vi "LSMcontroller_v62_updatedpointscan.vi"() -> ()   [LabVIEW 2015] (continued)
                                tunnel: [w2766 w2779] -> w2756
                                tunnel: w2760 -> [w2775 w2794]
                                tunnel: w2761 -> [w2765 w2785]
                                tunnel: w2762 -> [_ w2791]
                                frame False {
                                w2769 = u16 0 items=["unsigned binary", "offset binary", "2's complement"] ("data format (offset binary)")
                                n482 = Initialize Array(sgl 0.0, w2765) -> (w2772:sgl[])
                                n483 = Replace Array Subset(array=w2772, new element=sgl 1.0, index=0) -> (w2770:sgl[])
                                n484 = Reciprocal(x=w2775) -> (1/x=w2776:sgl)
                                n485 = Bundle By Name("Y"=w2770, "dt"=w2776) -> (w2767:waveform(sgl))  [unwired: 1 in]
                                n486 = call-poly <vilib>:"Analog to Digital.vi"("data format (offset binary)"=w2769, "compress digital (T)"=TRUE, "full-scale range (pk-pk)"=1.0, "resolution (16 bit)"=1, "analog waveform"=w2767) -> ("digital waveform"=w2766:digitalwaveform)  [unwired: 3 in, 3 out]
                                }
                                frame True {
                                w2782 = u16 0 items=["unsigned binary", "offset binary", "2's complement"] ("data format (offset binary)")
                                n487 = To Double Precision Float(number=w2785) -> (double precision float=w2792:dbl)
                                n488 = Initialize Array(sgl 0.0, w2785) -> (w2787:sgl[])
                                n489 = Divide(x=w2791, y=w2792) -> (x/y=w2789:dbl)
                                n490 = Round Toward +Infinity(x=w2789) -> (ceil(x): smallest int >= x=w2790:dbl)
                                n491 = Replace Array Subset(array=w2787, new element=sgl 1.0, index=0) -> (w2784:sgl[])
                                n492 = for {
                                N: w2790 -> [_]
                                tunnel: w2784 -> [w2796]
                                tunnel: [w2796] -> w2793 mode=concatenating
                                }
                                n493 = Reciprocal(x=w2794) -> (1/x=w2795:sgl)
                                n494 = Bundle By Name("Y"=w2793, "dt"=w2795) -> (w2780:waveform(sgl))  [unwired: 1 in]
                                n495 = call-poly <vilib>:"Analog to Digital.vi"("data format (offset binary)"=w2782, "compress digital (T)"=TRUE, "full-scale range (pk-pk)"=1.0, "resolution (16 bit)"=1, "analog waveform"=w2780) -> ("digital waveform"=w2779:digitalwaveform)  [unwired: 3 in, 3 out]
                                }
                                }
                                n496 = Build Array (concatenate)(w2754, w2756) -> (w2752:digitalwaveform[])
                                n497 = call "waveformsDObuffer.vi"("DO wf in"=w2752, "command"="set") -> ()  [unwired: 1 out]
                                }
                                frame 2 {
                                n498 = call "waveformsDObuffer.vi"("command"="get") -> ("DO wf out"=w2800:digitalwaveform[])  [unwired: 1 in]
                                n499 = Delete From Array(array=w2800, length=1, index=w2803) -> (deleted portion=w2798:digitalwaveform[], array with subset deleted=w2797:digitalwaveform[])
                                n500 = call "waveformsDObuffer.vi"("DO wf in"=w2797, "command"="set") -> ()  [unwired: 1 out]
                                }
                                frame 3, Default {
                                }
                                frame 0 {
                                n501 = local read "Measurement"() -> (w2806:T4)
                                n502 = To Unsigned Long Integer(number=w2806) -> (unsigned 32bit integer=w2805:u32)
                                n503 = case shown="5..7" w2805 {
                                tunnel: w2807 -> [_ w2810]
                                tunnel: [_ w2809] -> w2804
                                frame 0..4, Default {
                                }
                                frame 5..7 {
                                n504 = call "2pparameters.vi"("command"="get") -> ("params out"=w2817:T10)  [unwired: 1 in]
                                n505 = Unbundle By Name(w2817) -> ("wavdet"=w2818:bool, "sAOxy"=w2820:i32, "refwfsize"=w2821:dbl, "srate Img"=w2819:sgl)
                                n506 = call "waveformsDObuffer.vi"("command"="get") -> ("DO wf out"=w2811:digitalwaveform[])  [unwired: 1 in]
                                n507 = Index Array(array=w2811, index=w2810) -> (element=w2812:digitalwaveform)
                                n508 = case shown="True" w2818 {
                                tunnel: [w2825 w2838] -> w2815
                                tunnel: w2819 -> [w2834 w2853]
                                tunnel: w2820 -> [w2824 w2844]
                                tunnel: w2821 -> [_ w2850]
                                frame False {
                                w2828 = u16 0 items=["unsigned binary", "offset binary", "2's complement"] ("data format (offset binary)")
                                n509 = Initialize Array(sgl 0.0, w2824) -> (w2831:sgl[])
                                n510 = Replace Array Subset(array=w2831, new element=sgl 1.0, index=0) -> (w2829:sgl[])
                                n511 = Reciprocal(x=w2834) -> (1/x=w2835:sgl)
                                n512 = Bundle By Name("Y"=w2829, "dt"=w2835) -> (w2826:waveform(sgl))  [unwired: 1 in]
                                n513 = call-poly <vilib>:"Analog to Digital.vi"("data format (offset binary)"=w2828, "compress digital (T)"=TRUE, "full-scale range (pk-pk)"=1.0, "resolution (16 bit)"=1, "analog waveform"=w2826) -> ("digital waveform"=w2825:digitalwaveform)  [unwired: 3 in, 3 out]
                                }
                                frame True {
                                w2841 = u16 0 items=["unsigned binary", "offset binary", "2's complement"] ("data format (offset binary)")
                                n514 = To Double Precision Float(number=w2844) -> (double precision float=w2851:dbl)
                                n515 = Initialize Array(sgl 0.0, w2844) -> (w2846:sgl[])
                                n516 = Divide(x=w2850, y=w2851) -> (x/y=w2848:dbl)
                                n517 = Round Toward +Infinity(x=w2848) -> (ceil(x): smallest int >= x=w2849:dbl)
                                n518 = Replace Array Subset(array=w2846, new element=sgl 1.0, index=0) -> (w2843:sgl[])
                                n519 = for {
                                N: w2849 -> [_]
                                tunnel: w2843 -> [w2855]
                                tunnel: [w2855] -> w2852 mode=concatenating
                                }
                                n520 = Reciprocal(x=w2853) -> (1/x=w2854:sgl)
                                n521 = Bundle By Name("Y"=w2852, "dt"=w2854) -> (w2839:waveform(sgl))  [unwired: 1 in]
                                n522 = call-poly <vilib>:"Analog to Digital.vi"("data format (offset binary)"=w2841, "compress digital (T)"=TRUE, "full-scale range (pk-pk)"=1.0, "resolution (16 bit)"=1, "analog waveform"=w2839) -> ("digital waveform"=w2838:digitalwaveform)  [unwired: 3 in, 3 out]
                                }
                                }
                                n523 = Build Array(w2812) -> (w2809:digitalwaveform[])
                                n524 = Replace Array Subset(array=w2811, new element=w2815, index=w2810) -> (w2808:digitalwaveform[])
                                n525 = call "waveformsDObuffer.vi"("DO wf in"=w2808, "command"="set") -> ()  [unwired: 1 out]
                                }
                                }
                                }
                                }
                              }
                              frame #10 {
                                n526 = local read "Meastab"() -> (w2870:enum32{"X-Y Image", "Linescan", "Timetrace"})
                                n527 = property on="refwf" class="Ring (strict)"() -> ("RingText.Text"=w2867:string)  [unwired: 2 in, 2 out]
                                n528 = case shown="\"Timetrace\"" w2870 {
                                tunnel: [w2872 w2873] -> w2871
                                frame "X-Y Image", Default {
                                n529 = local read "Sampling rate"() -> (w2872:dbl)
                                }
                                frame "Timetrace" {
                                n530 = local read "srateAODOtt"() -> (w2873:dbl)
                                }
                                }
                                n531 = call "waveformsAObuffer.vi"("command"="get") -> ("AO wf out"=w2858:waveform(dbl)[])  [unwired: 1 in]
                                n532 = local read "wavdet"() -> (w2868:bool)
                                n533 = call "waveformsDObuffer.vi"("command"="get") -> ("DO wf out"=w2862:digitalwaveform[])  [unwired: 1 in]
                                n534 = call "correctwaveformsizetemp.vi"("new sampling frequency (Hz)"=w2871, "start"=TRUE, "reference waveforms to"=w2867, "Analog waveforms in"=w2858, "stop"=FALSE, "Digital waveforms in"=w2862) -> ("analog wf out"=w2864:waveform(dbl)[], "Digital wf out"=w2866:digitalwaveform[], "measpoints"=w2869:i32)
                                n535 = call "GetNumCamFramesv2.vi"("Digital Waveform Graph"=w2866) -> ("Numeric"=w2865:i32)  [unwired: 10 in]
                                n536 = call "waveformsDObuffer.vi"("DO wf in"=w2866, "command"="set") -> ()  [unwired: 1 out]
                                n537 = call "waveformsAObuffer.vi"("AO wf in"=w2864, "command"="set") -> ()  [unwired: 1 out]
                                n538 = local write "Total Camera Frames"(w2865) -> ()
                                n539 = case shown="True" w2868 {
                                tunnel: w2869 -> [_ w2874]
                                frame False {
                                }
                                frame True {
                                n540 = local write "# of frames"(w2874) -> ()
                                }
                                }
                              }
                            }
                          }
                          frame #6 {
                            # "Disabled for conversion to 64 bit"
                            n541 = disable-structure shown="Disabled" {
                              frame Disabled {
                                n542 = local read "Measurement"() -> (w2879:T4)
                                n543 = case shown="\"Lifetime (scan)\"" w2879 {
                                frame "X-Y-t movie", Default {
                                }
                                frame "Lifetime (scan)" {
                                # "total acquisition time"
                                n544 = call "2pparameters.vi"("command"="get") -> ("params out"=w2885:T10)  [unwired: 1 in]
                                n545 = Unbundle By Name(w2885) -> ("measpoints"=w2906:i32, "avpp"=w2907:i32, "sAOxy"=w2886:i32, "srate Img"=w2908:sgl)
                                n546 = Multiply(x=w2906, y=w2907) -> (x*y=w2904:i32)
                                n547 = To Double Precision Float(number=w2886) -> (double precision float=w2891:dbl)
                                n548 = Divide(x=w2891, y=w2908) -> (x/y=w2893:dbl)
                                n549 = To Double Precision Float(number=w2904) -> (double precision float=w2889:dbl)
                                n550 = local read "min phot"() -> (w2900:u32)
                                n551 = local read "expected c/s"() -> (w2901:dbl)
                                n552 = Multiply(x=w2889, y=w2893) -> (x*y=w2887:dbl)
                                n553 = Multiply(x=w2887, y=1000.0) -> (x*y=w2892:dbl)
                                n554 = local read "Ch1 ZeroX"() -> (w2898:i32)
                                n555 = local read "truncate"() -> (w2899:u32)
                                n556 = To Long Integer(number=w2892) -> (32bit integer=w2902:i32)
                                n557 = To Long Integer(number=w2901) -> (32bit integer=w2903:i32)
                                n558 = local read "Number of Bins"() -> (w2894:u32)
                                n559 = local read "Ch1 Level"() -> (w2896:i32)
                                n560 = local read "Ch0 ZeroX"() -> (w2897:i32)
                                n561 = local write "Acquisition time"(w2902) -> ()
                                n562 = local read "Ch0 Level"() -> (w2895:i32)
                                n563 = call "lifetimeparameters.vi"("command"="get") -> ("Params out"=w2883:T19)  [unwired: 1 in]
                                n564 = Add(x=10, y=w2902) -> (x+y=w2890:i32)
                                n565 = Bundle By Name(cluster=w2883, "acq time"=w2890, "acq rate"=w2903, "# bins"=w2894, "Ch0 Level"=w2895, "Ch1 Level"=w2896, "Ch0 ZeroX"=w2897, "Ch1 ZeroX"=w2898, "min photons"=w2900, "truncate"=w2899) -> (w2882:T19)
                                n566 = local write "Acquisition rate"(w2903) -> ()
                                n567 = call "lifetimeparameters.vi"("Params in"=w2882, "command"="set") -> ()  [unwired: 1 out]
                                }
                                }
                                n568 = local read "min phot"() -> (w2877:u32)
                                n569 = Decrement(x=w2877) -> (x-1=w2878:u32)
                                n570 = To Double Precision Float(number=w2878) -> (double precision float=w2876:dbl)
                                n571 = property on="img_CH1" class="IntGraph (strict)"("ZScale.Minimum"=w2876) -> ()  [unwired: 2 in, 2 out]
                              }
                              frame Enabled {
                              }
                            }
                            n572 = local write "64bit disabled"(TRUE ("64bit disabled")) -> ()
                          }
                          frame #7 {
                            n573 = local read "Sampling rate"() -> (w2910:dbl)
                            n574 = call "calcdaqtime.vi"("sampling rate"=w2910) -> ("Calc. time per frame (ms)"=w2909:dbl)
                            n575 = local write "Calc. time per frame (ms)"(w2909) -> ()
                          }
                          frame #8 {
                            n576 = call "2pparameters.vi"("command"="get") -> ("params out"=w2921:T10)  [unwired: 1 in]
                            n577 = local read "Measurement"() -> (w2912:T4)
                            n578 = Unbundle By Name(w2921) -> ("bufferAI"=w2919:i32, "srate"=w2920:sgl)
                            n579 = To Double Precision Float(number=w2919) -> (double precision float=w2913:dbl)
                            n580 = To Double Precision Float(number=w2920) -> (double precision float=w2923:dbl)
                            n581 = case shown="\"X-Y-t movie\", Default" w2912 {
                              tunnel: [w2928 w2932] -> w2911
                              frame "X-Y-t movie", Default {
                                n582 = local read "wavdet"() -> (w2929:bool)
                                n583 = case shown="False" w2929 {
                                tunnel: [w2930 w2931] -> w2928
                                frame False {
                                w2930 = 10123 items=["Finite Samples"=10178, "Continuous Samples"=10123, "Hardware Timed Single Point"=12522] ("sample mode")
                                }
                                frame True {
                                w2931 = 10123 items=["Finite Samples"=10178, "Continuous Samples"=10123, "Hardware Timed Single Point"=12522] ("sample mode")
                                }
                                }
                              }
                              frame "X-Y-Z stack" {
                                w2932 = 10178 items=["Finite Samples"=10178, "Continuous Samples"=10123, "Hardware Timed Single Point"=12522] ("sample mode")
                              }
                            }
                            n584 = Divide(x=w2913, y=w2923) -> (x/y=w2927:dbl)
                            n585 = Multiply(x=w2927, y=2.0) -> (x*y=w2924:dbl)
                            n586 = Max & Min(x=w2924, y=10.0) -> (max(x,y)=w2914:dbl)  [unwired: 1 out]
                            n587 = call "2pparameters.vi"("command"="get") -> ("params out"=w2918:T10)  [unwired: 1 in]
                            n588 = Bundle By Name(cluster=w2918, "timeout"=w2914, "sample mode"=w2911) -> (w2915:T10)
                            n589 = call "2pparameters.vi"("Params in"=w2915, "command"="set") -> ()  [unwired: 1 out]
                          }
                          frame #9 {
                            n590 = local read "# of frames"() -> (w2933:i32)
                            n591 = call "timestamps.vi"("# of frames"=w2933, "command"="init") -> ()  [unwired: 2 in, 1 out]
                          }
                        }
                      }
                      frame #2 {
                        # "Disabled for conversion to 64 bit"
                        n592 = call "prepAO_img.vi"() -> ("Terminal Name with Device Prefix"=w2936:tag)
                        n593 = call "prepAI_img.vi"("triggersource"=w2936) -> ()  [unwired: 2 in]
                        n594 = call "prepCI_img.vi"("ArmStart.DigEdge.Src"=w2936) -> ()  [unwired: 1 in]
                        n595 = call "prepDO_img.vi"() -> ()  [unwired: 2 in]
                        n596 = disable-structure shown="Disabled" {
                          frame Disabled {
                            n597 = local read "Measurement"() -> (w2937:T4)
                            n598 = case shown="\"Lifetime (scan)\"" w2937 {
                              frame "X-Y-t movie", Default {
                              }
                              frame "Lifetime (scan)" {
                                n599 = stacked-sequence {
                                frame #0 {
                                n600 = call "PH-temp.vi"("String"="clear" ("command")) -> ()  [unwired: 2 in, 2 out]
                                n601 = call "PH-temp-raw.vi"("command"="empty") -> ()  [unwired: 1 in, 1 out]
                                }
                                frame #1 {
                                n602 = call "calib.vi"() -> ()  [unwired: 1 in]
                                }
                                frame #2 {
                                n603 = call "setup.vi"() -> ()  [unwired: 1 in]
                                }
                                }
                              }
                            }
                          }
                          frame Enabled {
                          }
                        }
                        n604 = local write "64bit disabled"(TRUE ("64bit disabled")) -> ()
                      }
                      frame #3 {
                        n605 = local read "save\ndata"() -> (w2940:bool)
                        n606 = case shown="True" w2940 {
                          tunnel: w2941 -> [_ w2945]
                          frame False {
                          }
                          frame True {
                            n607 = local read "filename prefix"() -> (w2943:string)
                            n608 = local read "data dir"() -> (w2944:path)
                            n609 = call "preparetiffs.vi"("filename prefix"=w2943, "data dir"=w2944, "timestamp"=w2945) -> ("full-filename"=w2942:string)  [unwired: 1 in]
                            n610 = local write "full-filename"(w2942) -> ()
                          }
                        }
                        n611 = call "preptempbuffers.vi"() -> ()  [unwired: 12 in]
                      }
                      frame #4 {
                        # "Disabled Thorlabs Zstage;\nneeds to be replaced by PI code"
                        n612 = local read "Measurement"() -> (w2946:T4)
                        n613 = case shown="\"X-Y-Z stack\"" w2946 {
                          frame "X-Y-t movie", Default {
                          }
                          frame "X-Y-Z stack" {
                            # "Move Z stage"
                            n614 = stacked-sequence {
                              seq-local: [w2948 _] -> [_ w2961]
                              frame #0 {
                                n615 = local read "Z-Start (um)"() -> (w2952:dbl)
                                n616 = local read "Z-end (um)"() -> (w2951:dbl)
                                n617 = local read "# of frames"() -> (w2953:i32)
                                n618 = call "calcZslice.vi"("current slice"=0, "# of Slices"=w2953, "Z-Start (um)"=w2952, "Z-end (um)"=w2951) -> ("zpos (V)"=w2949:dbl, "zpos (um)"=w2948:dbl)
                                n619 = call "moveZ_V2.vi"("Z"=w2949) -> ()
                                n620 = local write "Cal. Z"(w2948) -> ()
                              }
                              frame #1 {
                                n621 = local read "Pstart"() -> (w2960:dbl)
                                n622 = local read "Pend"() -> (w2959:dbl)
                                n623 = local read "exp?"() -> (w2958:bool)
                                n624 = local read "Z-Start (um)"() -> (w2963:dbl)
                                n625 = local read "Z0"() -> (w2964:dbl)
                                n626 = local read "Z-end (um)"() -> (w2962:dbl)
                                n627 = local read "wavelength(nm)"() -> (w2957:dbl)
                                n628 = local read "# of frames"() -> (w2956:i32)
                                n629 = call "pockelscellzstage.vi"("current slice"=0, "# of Slices"=w2956, "wavelength (nm)"=w2957, "Z0"=w2964, "exp?"=w2958, "Zstart"=w2963, "Pend"=w2959, "Pstart"=w2960, "Z"=w2961, "Zend"=w2962) -> ("T(%)"=w2954:dbl)  [unwired: 1 in]
                                n630 = property on="Laserpower \n(%)" class="Slide (strict)"("Value"=w2954) -> ()  [unwired: 2 in, 2 out]
                                n631 = property on="lpow" class="DigNum (strict)"("Value"=w2954) -> ()  [unwired: 2 in, 2 out]
                              }
                            }
                          }
                        }
                        n632 = local write "Thorlabs Zstage disabled"(TRUE ("64bit disabled")) -> ()
                      }
                      frame #5 {
                        n633 = flat-sequence {
                          frame #0 {
                            n634 = call "2pparameters.vi"("command"="get") -> ("params out"=w2966:T10)  [unwired: 1 in]
                            n635 = Unbundle By Name(w2966) -> ("autoshutter"=w2967:bool)
                            n636 = case shown="True" w2967 {
                              frame False {
                              }
                              frame True {
                                n637 = call "shuttercontrol.vi"("command"="open") -> ()  [unwired: 1 in, 1 out]
                              }
                            }
                          }
                          frame #1 {
                            n638 = call "2pparameters.vi"("command"="get") -> ("params out"=w2971:T10)  [unwired: 1 in]
                            n639 = Tick Count (ms)() -> (millisecond timer value=w2970:u32)
                            n640 = Bundle By Name(cluster=w2971, "starttick"=w2970) -> (w2969:T10)
                            n641 = call "2pparameters.vi"("Params in"=w2969, "command"="set") -> ()  [unwired: 1 out]
                          }
                        }
                      }
                      frame #6 {
                        n642 = local read "Measurement"() -> (w2974:T4)
                        n643 = case shown="\"Lifetime (scan)\"" w2974 {
                          frame "X-Y-t movie" {
                            n644 = flat-sequence {
                              frame #0 {
                                n645 = call "runAI_img.vi"() -> ()  [unwired: 12 in]
                                n646 = call "runCI.vi"() -> ()  [unwired: 12 in]
                                n647 = call "runDO_img.vi"() -> ()  [unwired: 12 in]
                              }
                              frame #1 {
                                n648 = call "runAO_img.vi"() -> ()  [unwired: 12 in]
                              }
                            }
                          }
                          frame "Lifetime (scan)" {
                            # "Disabled for conversion to 64 bit"
                            n649 = disable-structure shown="Disabled" {
                              frame Disabled {
                                n650 = flat-sequence {
                                frame #0 {
                                n651 = call "runLT_img.vi"() -> ()  [unwired: 1 in]
                                n652 = call "runDO_img.vi"() -> ()  [unwired: 12 in]
                                }
                                frame #1 {
                                n653 = call "runAI_img.vi"() -> ()  [unwired: 12 in]
                                n654 = call "runCI.vi"() -> ()  [unwired: 12 in]
                                }
                                frame #2 {
                                n655 = call "runAO_img.vi"() -> ()  [unwired: 12 in]
                                }
                                }
                              }
                              frame Enabled {
                              }
                            }
                            n656 = local write "64bit disabled"(TRUE ("64bit disabled")) -> ()
                          }
                          frame "X-Y-Z stack", Default {
                          }
                        }
                      }
                      frame #7 {
                        # "Disabled for conversion to 64 bit"
                        n657 = while {
                          i -> [w3003]
                          stop <- w3000 stop-if-true
                          n658 = local read "Exit"() -> (w3008:bool)
                          n659 = local read "Stop"() -> (w2999:bool)
                          n660 = Or(x=w2999, y=w3008) -> (x .or. y?=w3004:bool)
                          n661 = case shown="False" w3004 {
                            tunnel: w3003 -> [w3009 _]
                            frame False {
                              n662 = stacked-sequence {
                                seq-local: [w3011 _ _ _ _ _ _] -> [_ _ _ _ _ _ w3140]
                                seq-local: [w3010 _ _ _ _ _ _] -> [_ _ _ _ _ _ w3139]
                                tunnel: w3009 -> [_ w3017 _ _ _ _ _]
                                frame #0 {
                                n663 = local read "Live"() -> (w3012:bool)
                                n664 = case shown="True" w3012 {
                                tunnel: [_ w3014] -> w3011
                                tunnel: [_ w3013] -> w3010
                                frame False {
                                }
                                frame True {
                                n665 = local read "Laserpower \n(%)"() -> (w3013:dbl)
                                n666 = local read "lpow"() -> (w3014:dbl)
                                }
                                }
                                n667 = call "preptempbuffers.vi"() -> ()  [unwired: 12 in]
                                }
                                frame #1 {
                                # "Move in Z if necessary"
                                # "Disabled Thorlabs Zstage;\nneeds to be replaced by PI code"
                                n668 = local read "Measurement"() -> (w3015:T4)
                                n669 = case shown="\"X-Y-Z stack\"" w3015 {
                                tunnel: w3017 -> [_ w3018]
                                frame "X-Y-t movie", Default {
                                }
                                frame "X-Y-Z stack" {
                                n670 = stacked-sequence {
                                seq-local: [w3019 _] -> [_ w3027]
                                tunnel: w3018 -> [w3021 w3026]
                                frame #0 {
                                n671 = local read "Z-Start (um)"() -> (w3023:dbl)
                                n672 = local read "Z-end (um)"() -> (w3022:dbl)
                                n673 = local read "# of frames"() -> (w3024:i32)
                                n674 = call "calcZslice.vi"("current slice"=w3021, "# of Slices"=w3024, "Z-Start (um)"=w3023, "Z-end (um)"=w3022) -> ("zpos (V)"=w3020:dbl, "zpos (um)"=w3019:dbl)
                                n675 = local write "Cal. Z"(w3019) -> ()
                                n676 = call "moveZ_V2.vi"("Z"=w3020) -> ()
                                }
                                frame #1 {
                                n677 = local read "Pstart"() -> (w3032:dbl)
                                n678 = local read "Pend"() -> (w3031:dbl)
                                n679 = local read "exp?"() -> (w3030:bool)
                                n680 = local read "Z-Start (um)"() -> (w3034:dbl)
                                n681 = local read "Z0"() -> (w3035:dbl)
                                n682 = local read "Z-end (um)"() -> (w3033:dbl)
                                n683 = local read "wavelength(nm)"() -> (w3029:dbl)
                                n684 = local read "# of frames"() -> (w3028:i32)
                                n685 = call "pockelscellzstage.vi"("current slice"=w3026, "# of Slices"=w3028, "wavelength (nm)"=w3029, "Z0"=w3035, "exp?"=w3030, "Zstart"=w3034, "Pend"=w3031, "Pstart"=w3032, "Z"=w3027, "Zend"=w3033) -> ("T(%)"=w3025:dbl)  [unwired: 1 in]
                                n686 = property on="Laserpower \n(%)" class="Slide (strict)"("Value"=w3025) -> ()  [unwired: 2 in, 2 out]
                                n687 = property on="lpow" class="DigNum (strict)"("Value"=w3025) -> ()  [unwired: 2 in, 2 out]
                                }
                                }
                                }
                                }
                                n688 = local write "Thorlabs Zstage disabled"(TRUE ("64bit disabled")) -> ()
                                }
                                frame #2 {
                                # "main loop"
                                n689 = for {
                                N: "avpp" -> [_]
                                i -> [w3041]
                                n690 = local read "Stop"() -> (w3039:bool)
                                n691 = local read "Exit"() -> (w3038:bool)
                                n692 = Increment(x=w3041) -> (x+1=w3040:i32)
                                n693 = Or(x=w3039, y=w3038) -> (x .or. y?=w3037:bool)
                                n694 = case shown="False" w3037 {
                                tunnel: w3040 -> [w3042 _]
                                frame False {
                                n695 = stacked-sequence {
                                seq-local: [w3043 _ _ _ _ _ _] -> [_ _ _ w3056 w3068 w3076 _]
                                tunnel: w3042 -> [w3044 _ _ _ _ _ _]
                                frame #0 {
                                n696 = local read "Live"() -> (w3043:bool)
                                n697 = case shown="True" w3043 {
                                tunnel: w3044 -> [_ w3047]
                                frame False {
                                }
                                frame True {
                                # "collect timetag for current image\nplus curent average"
                                n698 = To Single Precision Float(number=w3047) -> (single precision float=w3045:sgl)
                                n699 = Tick Count (ms)() -> (millisecond timer value=w3046:u32)
                                n700 = local write "Tick for Frame"(w3046) -> ()
                                n701 = local write "Current Average"(w3045) -> ()
                                }
                                }
                                }
                                frame #1 {
                                n702 = local read "Measurement"() -> (w3048:T4)
                                n703 = case shown="\"X-Y-Z stack\"" w3048 {
                                frame "X-Y-t movie", Default {
                                }
                                frame "X-Y-Z stack" {
                                n704 = stacked-sequence {
                                frame #0 {
                                n705 = disable-structure shown="Disabled" {
                                frame Disabled {
                                n706 = call "2pparameters.vi"("command"="get") -> ("params out"=w3050:T10)  [unwired: 1 in]
                                n707 = Unbundle By Name(w3050) -> ("autoshutter"=w3051:bool)
                                n708 = case shown="True" w3051 {
                                frame False {
                                }
                                frame True {
                                n709 = call "shuttercontrol.vi"("command"="open") -> ()  [unwired: 1 in, 1 out]
                                }
                                }
                                }
                                frame Enabled {
                                }
                                }
                                }
                                frame #1 {
                                n710 = call "runAI_img.vi"() -> ()  [unwired: 12 in]
                                n711 = call "runCI.vi"() -> ()  [unwired: 12 in]
                                n712 = call "runDO_img.vi"() -> ()  [unwired: 12 in]
                                }
                                frame #2 {
                                n713 = call "runAO_img.vi"() -> ()  [unwired: 12 in]
                                }
                                }
                                }
                                }
                                }
                                frame #2 {
                                n714 = call "collectCI_img.vi"() -> ("Avg cts/s"=w3055:dbl, "recorded samples"=w3054:i32)  [unwired: 1 out]
                                n715 = call "collectAI_img.vi"() -> ("wrap"=w3053:i32)  [unwired: 3 in]
                                n716 = local write "scol"(w3054) -> ()
                                n717 = local write "wrap"(w3053) -> ()
                                n718 = local write "Avg Counts/s"(w3055) -> ()
                                }
                                frame #3 {
                                n719 = case shown="True" w3056 {
                                frame False {
                                }
                                frame True {
                                n720 = local read "Measurement"() -> (w3057:T4)
                                n721 = case shown="\"X-Y-t movie\", Default" w3057 {
                                frame "X-Y-t movie", Default {
                                n722 = local read "ROI Type"() -> (w3058:u16)
                                n723 = case shown="0" w3058 {
                                frame 0 {
                                # "display chosen channels"
                                n724 = local read "Current Average"() -> (w3067:sgl)
                                n725 = local read "image1list"() -> (w3063:u16)
                                n726 = local read "image2list"() -> (w3066:u16)
                                n727 = To Unsigned Word Integer(number=w3066) -> (unsigned 16bit integer=w3061:u16)
                                n728 = To Unsigned Word Integer(number=w3063) -> (unsigned 16bit integer=w3062:u16)
                                n729 = call "dattoimage.vi"("image2list"=w3061, "Current Average"=w3067, "image1list"=w3062) -> ("image 2 array out"=w3065:sgl[][], "image 1 array out"=w3064:sgl[][])
                                n730 = Transpose 2D Array(2D array=w3064) -> (transposed array=w3060:sgl[][])
                                n731 = Transpose 2D Array(2D array=w3065) -> (transposed array=w3059:sgl[][])
                                n732 = local write "img_CH1"(w3060) -> ()
                                n733 = local write "img_CH2"(w3059) -> ()
                                }
                                frame 1, Default {
                                }
                                }
                                }
                                frame "Lifetime (scan)" {
                                }
                                }
                                }
                                }
                                }
                                frame #4 {
                                n734 = case shown="True" w3068 {
                                frame False {
                                }
                                frame True {
                                # "set colormaps"
                                n735 = call "misc-global.vi"("command"="get") -> ("misc out"=w3072:cluster{"Colormaps":u32[][]})  [unwired: 1 in]
                                n736 = Unbundle By Name(w3072) -> ("Colormaps"=w3071:u32[][])
                                n737 = control-ref of="img_CH1"() -> (w3075:refnum<vi>)
                                n738 = control-ref of="img_CH2"() -> (w3074:refnum<vi>)
                                n739 = Index Array(array=w3071, index (row)="Colormap") -> (element=w3070:u32[])  [unwired: 1 in]
                                n740 = property class="IntGraph (strict)"(reference=w3075, "Color Table"=w3070) -> ()  [unwired: 1 in, 2 out]
                                n741 = property class="IntGraph (strict)"(reference=w3074, "Color Table"=w3070) -> ()  [unwired: 1 in, 2 out]
                                }
                                }
                                }
                                frame #5 {
                                n742 = case shown="True" w3076 {
                                frame False {
                                }
                                frame True {
                                # "crude estimate of time per frame\n(resolution is 1 ms), not so much for\nplotting purposes, more for debugging\ncollection and processing data"
                                n743 = local read "ypixels ref"() -> (w3081:i32)
                                n744 = local read "Tick for Frame"() -> (w3082:u32)
                                n745 = Tick Count (ms)() -> (millisecond timer value=w3083:u32)
                                n746 = To Double Precision Float(number=w3081) -> (double precision float=w3080:dbl)
                                n747 = Subtract(x=w3083, y=w3082) -> (x-y=w3078:u32)
                                n748 = To Double Precision Float(number=w3078) -> (double precision float=w3079:dbl)
                                n749 = local write "Meas. time per frame (ms)"(w3078) -> ()
                                n750 = Divide(x=w3079, y=w3080) -> (x/y=w3077:dbl)
                                n751 = local write "time per line (ms)"(w3077) -> ()
                                }
                                }
                                }
                                frame #6 {
                                n752 = local read "Measurement"() -> (w3084:T4)
                                n753 = case shown="\"X-Y-Z stack\"" w3084 {
                                frame "X-Y-t movie", Default {
                                }
                                frame "X-Y-Z stack" {
                                n754 = call "2pparameters.vi"("command"="get") -> ("params out"=w3086:T10)  [unwired: 1 in]
                                n755 = Unbundle By Name(w3086) -> ("autoshutter"=w3087:bool)
                                n756 = call "stopCI_img.vi"() -> ()  [unwired: 12 in]
                                n757 = call "stopAI_img.vi"() -> ()  [unwired: 12 in]
                                n758 = case shown="True" w3087 {
                                frame False {
                                }
                                frame True {
                                n759 = call "shuttercontrol.vi"("command"="close") -> ()  [unwired: 1 in, 1 out]
                                }
                                }
                                n760 = Wait (ms)(milliseconds to wait=u32 100) -> ()  [unwired: 1 out]
                                n761 = call "stopAO_img.vi"() -> ()  [unwired: 12 in]
                                n762 = call "stopDO_img.vi"() -> ()  [unwired: 12 in]
                                }
                                }
                                }
                                }
                                }
                                frame True {
                                }
                                }
                                }
                                }
                                frame #3 {
                                n763 = local read "Measurement"() -> (w3090:T4)
                                n764 = case shown="\"Lifetime (scan)\"" w3090 {
                                frame "X-Y-t movie", Default {
                                }
                                frame "Lifetime (scan)" {
                                w3093 = u16 2 items=["Stream to disk", "Post process", "real time process"] ("Ring")
                                n765 = local read "T3R Data processing"() -> (w3094:u16)
                                n766 = Equal?(x=w3094, y=w3093) -> (x = y?=w3092:bool)
                                n767 = case shown="True" w3092 {
                                frame False {
                                }
                                frame True {
                                n768 = disable-structure shown="Disabled" {
                                frame Disabled {
                                n769 = local read "lineshift"() -> (w3097:i32)
                                n770 = call "wrapcutlifetime.vi"("lineshift"=w3097) -> ("pt3img"=w3099:u16[][], "lifetimes"=w3098:sgl[][], "okay"=w3095:bool, "# of frames"=w3096:i32)
                                n771 = case shown="True" w3095 {
                                tunnel: w3099 -> [_ w3109]
                                tunnel: w3098 -> [_ w3107]
                                tunnel: w3096 -> [_ w3103]
                                frame False {
                                }
                                frame True {
                                # "lifetime"
                                # "intensity"
                                n772 = Transpose 2D Array(2D array=w3109) -> (transposed array=w3101:u16[][])
                                n773 = Transpose 2D Array(2D array=w3107) -> (transposed array=w3108:sgl[][])
                                n774 = local write "frames recorded"(w3103) -> ()
                                n775 = local read "counts"() -> (w3102:i32)
                                n776 = Array Max & Min(array=w3101) -> (max value=w3106:u16)  [unwired: 3 out]
                                n777 = To Single Precision Float(number=w3101) -> (single precision float=w3100:sgl[][])
                                n778 = local write "img_CH2"(w3108) -> ()
                                n779 = local write "img_CH1"(w3100) -> ()
                                n780 = Quotient & Remainder(x=w3102, y=w3103) -> (floor(x/y)=→"photons/frame":i32)  [unwired: 1 out]
                                n781 = To Double Precision Float(number=w3106) -> (double precision float=w3105:dbl)
                                n782 = property on="img_CH1" class="IntGraph (strict)"("ZScale.Maximum"=w3105) -> ()  [unwired: 2 in, 2 out]
                                }
                                }
                                }
                                frame Enabled {
                                }
                                }
                                }
                                }
                                }
                                }
                                n783 = local read "save\ndata"() -> (w3091:bool)
                                n784 = case shown="True" w3091 {
                                frame False {
                                }
                                frame True {
                                n785 = local read "Current Average"() -> (w3110:sgl)
                                n786 = call "savetiffs.vi"("current average"=w3110) -> ()
                                }
                                }
                                }
                                frame #4 {
                                n787 = local read "save\ndata"() -> (w3111:bool)
                                n788 = case shown="True" w3111 {
                                frame False {
                                }
                                frame True {
                                n789 = local read "points recorded"() -> (w3113:i32)
                                n790 = call "timestamps.vi"("points recorded"=w3113, "command"="add") -> ()  [unwired: 2 in, 1 out]
                                }
                                }
                                }
                                frame #5 {
                                n791 = local read "Live"() -> (w3114:bool)
                                n792 = case shown="True" w3114 {
                                frame False {
                                }
                                frame True {
                                n793 = local read "downright"() -> (w3119:bool)
                                n794 = local read "downleft"() -> (w3121:bool)
                                n795 = local read "upright"() -> (w3117:bool)
                                n796 = local read "upleft"() -> (w3115:bool)
                                n797 = local read "down"() -> (w3120:bool)
                                n798 = local read "right"() -> (w3118:bool)
                                n799 = local read "left"() -> (w3122:bool)
                                n800 = local read "up"() -> (w3116:bool)
                                n801 = Compound Arithmetic op=OR(w3115, w3116, w3117, w3118, w3119, w3120, w3121, w3122) -> (w3123:bool)
                                n802 = case shown="True" w3123 {
                                frame False {
                                }
                                frame True {
                                n803 = stacked-sequence {
                                frame #0 {
                                n804 = local read "downright"() -> (w3125:bool)
                                n805 = local read "downleft"() -> (w3127:bool)
                                n806 = local read "BigSmall"() -> (w3124:bool)
                                n807 = local read "upright"() -> (w3129:bool)
                                n808 = local read "upleft"() -> (w3132:bool)
                                n809 = local read "down"() -> (w3128:bool)
                                n810 = local read "right"() -> (w3130:bool)
                                n811 = local read "left"() -> (w3126:bool)
                                n812 = local read "up"() -> (w3131:bool)
                                n813 = call "movestageparams.vi"("command"="get") -> ("Params out"=w3135:T20)  [unwired: 1 in]
                                n814 = Bundle By Name(cluster=w3135, "upleft"=w3132, "up"=w3131, "upright"=w3129, "right"=w3130, "downright"=w3125, "down"=w3128, "downleft"=w3127, "left"=w3126, "Bigsmall"=w3124) -> (w3136:T20)
                                n815 = call "movestageparams.vi"("Params in"=w3136, "command"="set") -> ()  [unwired: 1 out]
                                }
                                frame #1 {
                                n816 = call "movestage.vi"() -> ()  [unwired: 12 in]
                                }
                                frame #2 {
                                w3137 = FALSE ("OK Button")
                                w3138 = FALSE ("OK Button")
                                n817 = property on="down" class="Bool (strict)"("Value"=w3138) -> ()  [unwired: 2 in, 2 out]
                                n818 = property on="up" class="Bool (strict)"("Value"=w3138) -> ()  [unwired: 2 in, 2 out]
                                n819 = property on="right" class="Bool (strict)"("Value"=w3138) -> ()  [unwired: 2 in, 2 out]
                                n820 = property on="left" class="Bool (strict)"("Value"=w3138) -> ()  [unwired: 2 in, 2 out]
                                n821 = property on="upright" class="Bool (strict)"("Value"=w3137) -> ()  [unwired: 2 in, 2 out]
                                n822 = property on="downleft" class="Bool (strict)"("Value"=w3137) -> ()  [unwired: 2 in, 2 out]
                                n823 = property on="downright" class="Bool (strict)"("Value"=w3137) -> ()  [unwired: 2 in, 2 out]
                                n824 = property on="upleft" class="Bool (strict)"("Value"=w3137) -> ()  [unwired: 2 in, 2 out]
                                }
                                }
                                }
                                }
                                }
                                }
                                }
                                frame #6 {
                                n825 = local read "Live"() -> (w3141:bool)
                                n826 = case shown="True" w3141 {
                                tunnel: w3140 -> [_ w3148]
                                tunnel: w3139 -> [_ w3147]
                                frame False {
                                }
                                frame True {
                                n827 = local read "Laserpower \n(%)"() -> (w3143:dbl)
                                n828 = local read "lpow"() -> (w3142:dbl)
                                n829 = Not Equal?(x=w3142, y=w3148) -> (x != y?=w3144:bool)
                                n830 = Not Equal?(x=w3143, y=w3147) -> (x != y?=w3145:bool)
                                n831 = Or(x=w3145, y=w3144) -> (x .or. y?=w3146:bool)
                                n832 = case shown="True" w3146 {
                                tunnel: w3145 -> [_ w3152]
                                tunnel: w3144 -> [_ w3151]
                                tunnel: w3143 -> [_ w3150]
                                tunnel: w3142 -> [_ w3149]
                                frame False {
                                }
                                frame True {
                                n833 = case shown="True" w3152 {
                                tunnel: w3150 -> [_ w3155]
                                frame False {
                                }
                                frame True {
                                n834 = local read "wavelength(nm)"() -> (w3156:dbl)
                                n835 = call "setpockelscellT.vi"("wavelength(nm)"=w3156, "transmission"=w3155) -> ()  [unwired: 1 in]
                                n836 = property on="lpow" class="DigNum (strict)"("Value"=w3155) -> ()  [unwired: 2 in, 2 out]
                                }
                                }
                                n837 = case shown="True" w3151 {
                                tunnel: w3149 -> [_ w3153]
                                frame False {
                                }
                                frame True {
                                n838 = local read "wavelength(nm)"() -> (w3154:dbl)
                                n839 = call "setpockelscellT.vi"("wavelength(nm)"=w3154, "transmission"=w3153) -> ()  [unwired: 1 in]
                                n840 = property on="Laserpower \n(%)" class="Slide (strict)"("Value"=w3153) -> ()  [unwired: 2 in, 2 out]
                                }
                                }
                                }
                                }
                                }
                                }
                                }
                              }
                            }
                            frame True {
                            }
                          }
                          n841 = Increment(x=w3003) -> (x+1=w3002:i32)
                          "points recorded" <- w3002
                          n842 = call "stopcond.vi"("prec"=w3002) -> ("stop"=w3001:bool)
                          n843 = local read "Stop"() -> (w3007:bool)
                          n844 = local read "Exit"() -> (w3006:bool)
                          n845 = Or(x=w3007, y=w3006) -> (x .or. y?=w3005:bool)
                          n846 = Or(x=w3001, y=w3005) -> (x .or. y?=w3000:bool)
                        }
                        n847 = disable-structure shown="Disabled" {
                          disable-tunnel: w2977 -> [w2983 _]
                          frame Disabled {
                            w2980 = u16 0 items=["Stream to disk", "Post process", "real time process"] ("Ring")
                            n848 = local read "T3R Data processing"() -> (w2979:u16)
                            n849 = Equal?(x=w2979, y=w2980) -> (x = y?=w2978:bool)
                            n850 = local read "save\ndata"() -> (w2982:bool)
                            n851 = local read "Measurement"() -> (w2984:T4)
                            n852 = And(x=w2982, y=w2978) -> (x .and. y?=w2981:bool)
                            n853 = case shown="\"Lifetime (scan)\"" w2984 {
                              tunnel: w2983 -> [_ w2988]
                              tunnel: w2981 -> [_ w2987]
                              frame "X-Y-t movie", Default {
                              }
                              frame "Lifetime (scan)" {
                                n854 = case shown="True" w2987 {
                                selector: w2987 -> [w2989 w2994]
                                tunnel: w2988 -> [_ w2992]
                                tunnel: [path "" ("appended path") w2995] -> w2986
                                tunnel: [w2989 w2994] -> w2985
                                frame False {
                                }
                                frame True {
                                n855 = local read "filename prefix"() -> (w2993:string)
                                n856 = local read "data dir"() -> (w2996:path)
                                n857 = call "generatedatafilename.vi"("timestamp"=w2992, "filename prefix in"=w2993) -> ("full-filename"=w2991:string)
                                n858 = Concatenate Strings(w2991, ".lvpt3img" ("string")) -> (w2998:string)
                                n859 = Build Path(base path=w2996, name or relative path=w2998) -> (appended path=w2995:path)
                                }
                                }
                                n860 = call "collectLT_img_v2.vi"("stream?"=w2985, "data file"=w2986) -> ()  [unwired: 2 out]
                              }
                            }
                          }
                          frame Enabled {
                          }
                        }
                        n861 = local write "64bit disabled"(TRUE ("64bit disabled")) -> ()
                      }
                      frame #8 {
                        # "Disabled for conversion to 64 bit"
                        n862 = local read "Measurement"() -> (w3159:T4)
                        n863 = case shown="\"Lifetime (scan)\"" w3159 {
                          tunnel: w3158 -> [_ _ w3160]
                          frame "X-Y-t movie", Default {
                          }
                          frame "X-Y-Z stack" {
                            n864 = call "eraseDO_img.vi"() -> ()  [unwired: 12 in]
                            n865 = call "eraseAO_img.vi"() -> ()  [unwired: 12 in]
                            n866 = call "eraseCI_img.vi"() -> ()  [unwired: 12 in]
                            n867 = call "eraseAI_img.vi"() -> ()  [unwired: 12 in]
                          }
                          frame "Lifetime (scan)" {
                            n868 = disable-structure shown="Disabled" {
                              disable-tunnel: w3160 -> [w3161 _]
                              frame Disabled {
                                n869 = stacked-sequence {
                                tunnel: w3161 -> [_ _ w3175 _ _]
                                frame #0 {
                                n870 = disable-structure shown="Disabled" {
                                frame Disabled {
                                n871 = call "stoperaseCI.vi"() -> ()  [unwired: 12 in]
                                n872 = call "stoperaseDO_img.vi"() -> ()  [unwired: 12 in]
                                n873 = call "stoperaseAO_img.vi"() -> ()  [unwired: 12 in]
                                n874 = call "stoperaseAI_img.vi"() -> ()  [unwired: 12 in]
                                }
                                frame Enabled {
                                }
                                }
                                }
                                frame #1 {
                                n875 = disable-structure shown="Disabled" {
                                frame Disabled {
                                n876 = local read "Acquisition time"() -> (w3165:i32)
                                n877 = call "collect_allLT_img.vi"() -> ("counts"=w3167:i32)  [unwired: 1 out]
                                n878 = local read "counts"() -> (w3168:i32)
                                n879 = Add(x=w3168, y=w3167) -> (x+y=w3166:i32)
                                "counts" <- w3166
                                n880 = Divide(x=w3166, y=w3165) -> (x/y=w3164:dbl)
                                n881 = Multiply(x=1000.0, y=w3164) -> (x*y=w3163:dbl)
                                n882 = local write "Avg Counts/s"(w3163) -> ()
                                }
                                frame Enabled {
                                }
                                }
                                }
                                frame #2 {
                                w3171 = u16 0 items=["Stream to disk", "Post process", "real time process"] ("Ring")
                                n883 = local read "T3R Data processing"() -> (w3170:u16)
                                n884 = local read "save\ndata"() -> (w3173:bool)
                                n885 = Equal?(x=w3170, y=w3171) -> (x = y?=w3169:bool)
                                n886 = Not(x=w3169) -> (.not. x?=w3174:bool)
                                n887 = And(x=w3173, y=w3174) -> (x .and. y?=w3172:bool)
                                n888 = case shown="True" w3172 {
                                tunnel: w3175 -> [_ w3177]
                                frame False {
                                }
                                frame True {
                                n889 = local read "filename prefix"() -> (w3178:string)
                                n890 = local read "data dir"() -> (w3183:path)
                                n891 = call "2pparameters.vi"("command"="get") -> ("params out"=w3198:T10)  [unwired: 1 in]
                                n892 = call "generatedatafilename.vi"("timestamp"=w3177, "filename prefix in"=w3178) -> ("full-filename"=w3176:string)
                                n893 = Unbundle By Name(w3198) -> ("srate"=w3196:sgl, "sAOxy"=w3195:i32, "Xpixels Img"=w3193:i32, "Ypixels Img"=w3191:i32)
                                n894 = Concatenate Strings(w3176, ".lvpt3img" ("string")) -> (w3181:string)
                                n895 = Build Path(base path=w3183, name or relative path=w3181) -> (appended path=w3180:path)
                                n896 = To Unsigned Long Integer(number=w3196) -> (unsigned 32bit integer=w3197:u32)
                                n897 = To Unsigned Long Integer(number=w3195) -> (unsigned 32bit integer=w3194:u32)
                                n898 = To Unsigned Long Integer(number=w3193) -> (unsigned 32bit integer=w3192:u32)
                                n899 = To Unsigned Long Integer(number=w3191) -> (unsigned 32bit integer=w3190:u32)
                                n900 = call "PH-temp-raw.vi"("command"="get") -> ("array out"=w3189:u32[])  [unwired: 1 in]
                                n901 = Build Array (concatenate)(w3197, w3194, w3192, w3190, w3189) -> (w3188:u32[])
                                n902 = Open/Create/Replace File(file path (use dialog)=w3180, operation (0:open)=T8."replace or create") -> (refnum out=w3187:refnum<file>, error out=w3186:errorcluster)  [unwired: 4 in, 1 out]
                                n903 = Write to Binary File(file (use dialog)=w3187, data=w3188, error in=w3186, 5:FALSE ("prepend array or string size? (T)")) -> (refnum out=w3184:refnum<file>, error out=w3185:errorcluster)  [unwired: 2 in, 1 out]
                                n904 = Close File(refnum=w3184, error in=w3185) -> ()  [unwired: 2 out]
                                }
                                }
                                n905 = call "stoperaseLT_img.vi"() -> ()  [unwired: 1 in]
                                }
                                frame #3 {
                                w3204 = u16 1 items=["Stream to disk", "Post process", "real time process"] ("Ring")
                                n906 = local read "T3R Data processing"() -> (w3203:u16)
                                n907 = Equal?(x=w3203, y=w3204) -> (x = y?=w3202:bool)
                                n908 = case shown="True" w3202 {
                                frame False {
                                }
                                frame True {
                                # "intensity"
                                # "lifetime"
                                # "intensity"
                                n909 = property on="img_CH1" class="IntGraph (strict)"() -> ("Value"=w3217:sgl[][])  [unwired: 2 in, 2 out]
                                n910 = Array Max & Min(array=w3217) -> (max value=w3218:sgl)  [unwired: 3 out]
                                n911 = local read "lineshift"() -> (w3205:i32)
                                n912 = local read "min phot"() -> (w3219:u32)
                                n913 = To Unsigned Long Integer(number=w3218) -> (unsigned 32bit integer=w3221:u32)
                                n914 = local read "counts"() -> (w3207:i32)
                                n915 = call "wrapcutlifetime.vi"("lineshift"=w3205) -> ("pt3img"=w3216:u16[][], "lifetimes"=w3214:sgl[][], "okay"=w3209:bool, "# of frames"=w3206:i32)
                                "frames recorded" <- w3206
                                n916 = Greater?(x=w3219, y=w3221) -> (0:w3220:bool)
                                n917 = Quotient & Remainder(x=w3207, y=w3206) -> (floor(x/y)=w3208:i32)  [unwired: 1 out]
